vi "ListenCondensorMic.vi"() -> ()   [LabVIEW 2017]
uses:
  <vilib>/express/express analysis/Spectral/Block/exnSpectralBlock spectral measurements power poly.vi
  <vilib>/express/express analysis/Spectral/Block/exnSpectralBlock spectral measurements power DDT.vi
  <vilib>/express/express analysis/Spectral/XNode/ExpressSpectralMeasurementsBlockNode.xnode
panel:
  out "Complete":bool
  out "Listening":bool
  out "Raw Microphone Data":dynamicdata(graph)
  out "Power Spectrum":dynamicdata(graph)
  in  "Time (sec)":dbl(knob)=30.0 min=0.0 max=60.0 step=1.0 scale=0.0..60.0 scale format="%#_2g"
  in  "Analog Acquisition  2":cluster{"Analog Fs":u32}={"Analog Fs"=200000} {"Analog Fs" format="%0.0f"}
  in  "Device Name":tag="Dev2"
  in  "File Path":path=path "C:/Users/klt8/Documents"
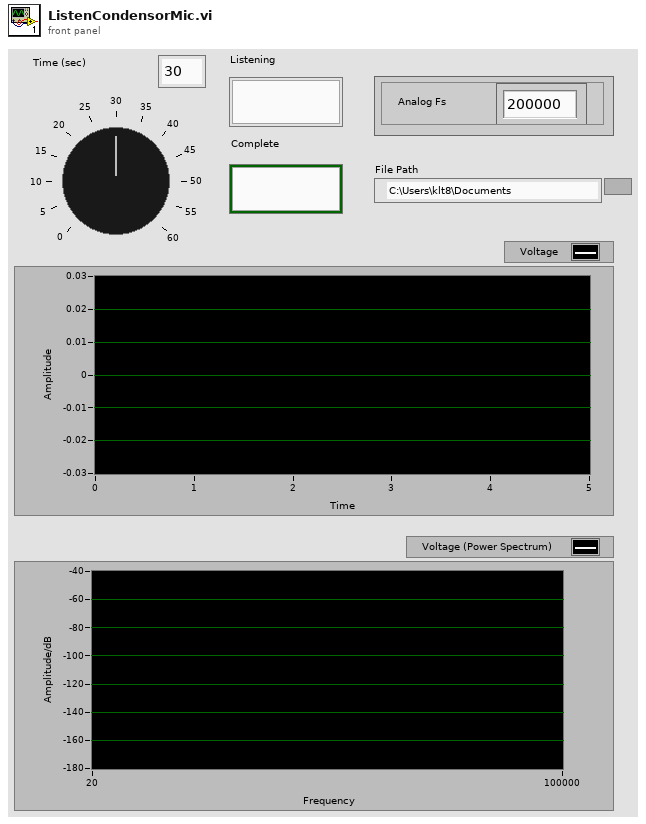
[diagram p1: front panel]
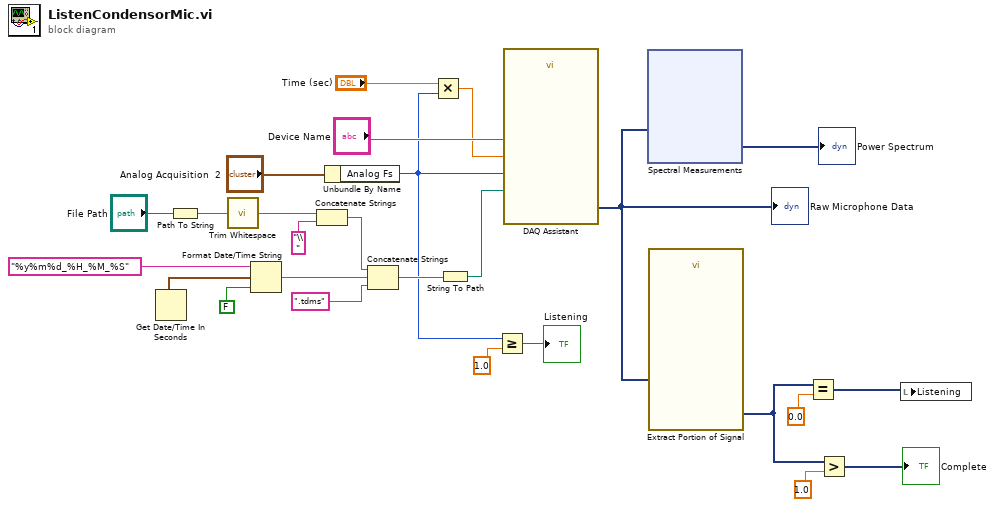
[diagram p0: block diagram]
diagram:
  n1 = Get Date/Time In Seconds() -> (seconds since 1Jan1904=w17:timestamp)
  n2 = Path To String(path="File Path") -> (string=w19:string)
  n3 = call <vilib>:"Trim Whitespace.vi"("string"=w19) -> ("trimmed string"=w20:string)  [unwired: 1 in]
  n4 = Format Date/Time String(time format string (%c)="%y%m%d_%H_%M_%S", seconds (now)=w17, UTC format=FALSE) -> (date/time string=w21:string)
  n5 = Concatenate Strings(w20, "\\" ("string")) -> (w13:string)
  n6 = Unbundle By Name("Analog Acquisition  2") -> ("Analog Fs"=w7:u32)
  n7 = Concatenate Strings(w13, w21, ".tdms" ("string")) -> (w11:string)
  n8 = Multiply(x="Time (sec)", y=w7) -> (x*y=w23:dbl)
  n9 = String To Path(string=w11) -> (path=w10:path)
  n10 = Greater Or Equal?(x=w7, y=1.0) -> (x >= y?=→"Listening":bool)
  n11 = call "DAQ Assistant"("rate"=w7, "number of samples"=w23, "file path"=w10, "device name"="Device Name") -> ("data"=w9:dynamicdata)  [unwired: 13 in, 2 out]
  "Raw Microphone Data" <- w9
  n12 = xnode "Spectral Measurements"("Signals"=w9) -> ("Power Spectrum"=→"Power Spectrum":dynamicdata)  [unwired: 1 in, 1 out]
  n13 = call "Extract Portion of Signal"("Signals"=w9) -> ("Section"=w1:dynamicdata)  [unwired: 9 in, 1 out]
  n14 = Equal?(x=w1, y=0.0 ("x")) -> (x = y?=w4:dynamicdata)
  n15 = Greater?(x=w1, y=1.0) -> (0:→"Complete":dynamicdata)
  n16 = local write "Listening"(w4) -> ()
